vi "_PC_MS_SubVI dataProcess.vi"(7 "Init?(F)":bool, 8 "error in (no error)":errorcluster, 10 "newSigInfo":T1, 11 "Reference":T2) -> (0 "error out":errorcluster, 3 "ydata":sgl[][](array[numeric]))   [LabVIEW 2018]
uses:
  <vilib>/Utility/miscctls.llb/LVPositionTypeDef.ctl
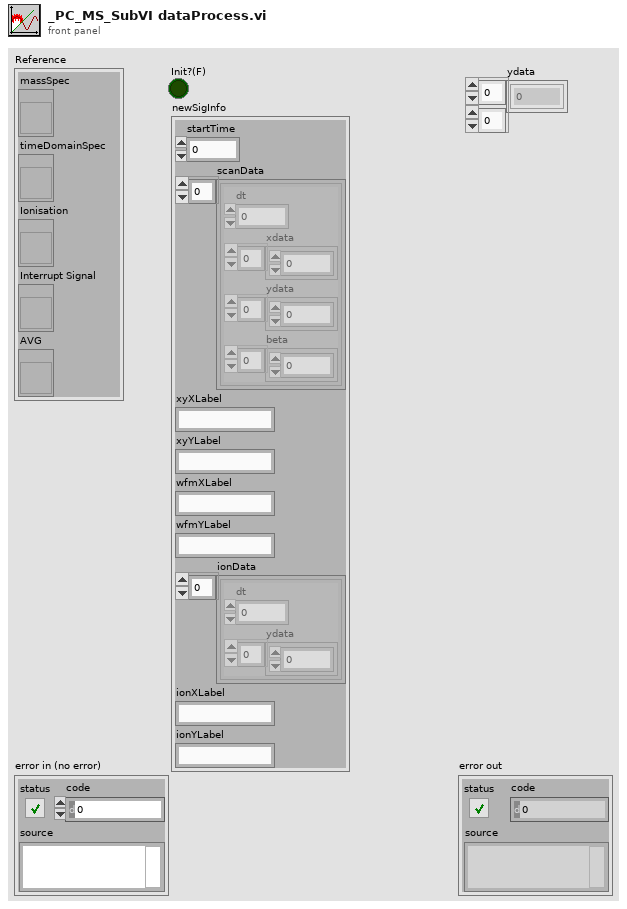
[diagram p1: front panel]
types:
  T1 = cluster{"startTime":dbl, "scanData":cluster{"dt":dbl, "xdata":dbl[], "ydata":sgl[], "beta":dbl[]}[], "xyXLabel":string, "xyYLabel":string, "wfmXLabel":string, "wfmYLabel":string, "ionData":cluster{"dt":dbl, "ydata":sgl[]}[], "ionXLabel":string, "ionYLabel":string}
  T2 = cluster{"massSpec":refnum<vi>, "timeDomainSpec":refnum<vi>, "Ionisation":refnum<vi>, "Interrupt Signal":refnum<vi>, "AVG":refnum<vi>}
  T3 = cluster{"massSpec":refnum<vi>, "timeDomainSpec":refnum<vi>, "Ionisation":refnum<vi>}
  T4 = typedef "LVPositionTypeDef.ctl" = cluster{"Left":i32, "Top":i32}
  T5 = typedef "LVRectTypeDef.ctl" = cluster{"Left":i16, "Top":i16, "Right":i16, "Bottom":i16}
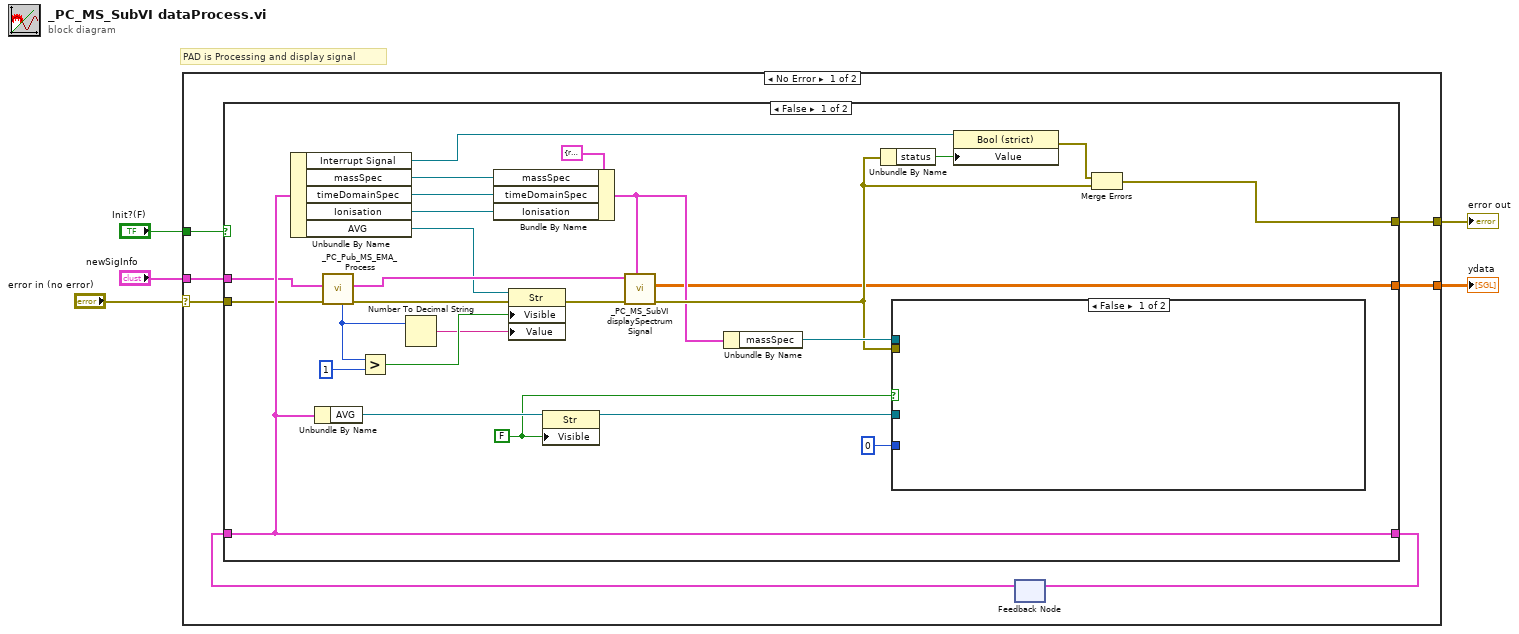
[diagram p0: block diagram]
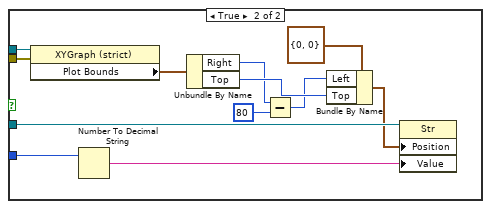
[diagram p2: hidden frame]
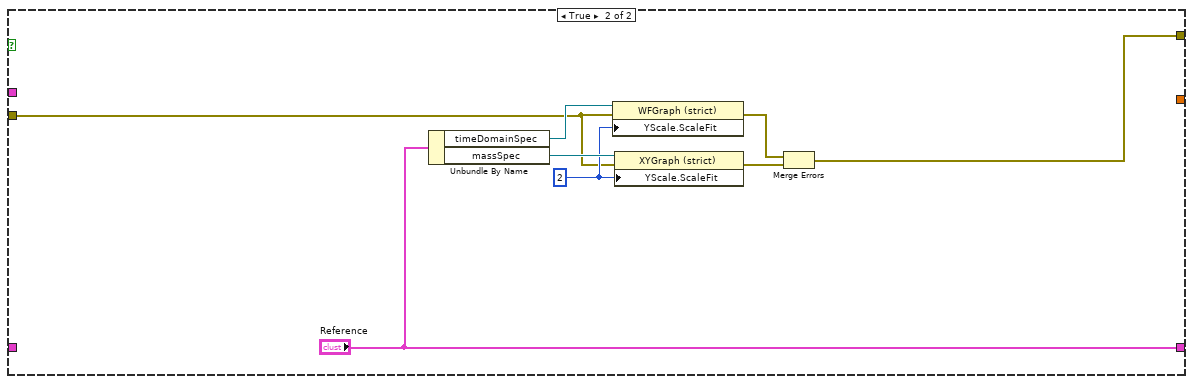
[diagram p3: hidden frame]
diagram:
  # "PAD is Processing and display signal"
  n1 = case shown="No Error" "error in (no error)" {
    selector: "error in (no error)" -> [w6 w60]
    tunnel: "Init?(F)" -> [w12 _]
    tunnel: [w11 w60] -> w4
    tunnel: "newSigInfo" -> [w8 _]
    tunnel: [w7 _] -> w2
    frame No Error {
      n2 = feedback #1() -> (w9:T2)  [unwired: 1 in]
      n3 = case shown="False" w12 {
        tunnel: w9 -> [w34 _]
        tunnel: [w34 "Reference"] -> w10
        tunnel: w8 -> [w22 _]
        tunnel: w6 -> [w20 w53]
        tunnel: [w36 w54] -> w11
        tunnel: [w23 _] -> w7
        frame False {
          w28 = FALSE ("Visible")
          n4 = Unbundle By Name(w34) -> ("Interrupt Signal"=w39:refnum<vi>, "massSpec"=w33:refnum<vi>, "timeDomainSpec"=w30:refnum<vi>, "Ionisation"=w26:refnum<vi>, "AVG"=w18:refnum<vi>)
          n5 = Unbundle By Name(w34) -> ("AVG"=w35:refnum<vi>)
          n6 = call "_PC_Pub_MS_EMA_Process.vi"("error in (no error)"=w20, "SigInfo in"=w22) -> ("error out"=w16:errorcluster, "SigInfo out"=w21:T1, "AVG Items"=w14:u8)  [unwired: 7 in]
          n7 = Greater?(x=w14, y=u8 1) -> (0:w17:bool)
          n8 = Number To Decimal String(number=w14) -> (decimal integer string=w13:string)  [unwired: 1 in]
          n9 = Bundle By Name(cluster=T3 {"massSpec"=refnum, "timeDomainSpec"=refnum, "Ionisation"=refnum}, "massSpec"=w33, "timeDomainSpec"=w30, "Ionisation"=w26) -> (w25:T3)
          n10 = property class="Str"(reference=w18, error in=w16, "Visible"=w17, "Value"=w13) -> (error out=w15:errorcluster)  [unwired: 1 out]
          n11 = property class="Str"(reference=w35, "Visible"=w28) -> (reference out=w37:refnum<vi>)  [unwired: 1 in, 1 out]
          n12 = call "_PC_MS_SubVI displaySpectrumSignal.vi"("graphRefnum in"=w25, "error in (no error)"=w15, "newSigInfo"=w21) -> ("error out"=w29:errorcluster, "ydata"=w23:sgl[][])  [unwired: 7 in]
          n13 = Unbundle By Name(w25) -> ("massSpec"=w32:refnum<vi>)
          n14 = Unbundle By Name(w29) -> ("status"=w38:bool)
          n15 = case shown="False" w28 {
            tunnel: w32 -> [_ w51]
            tunnel: w37 -> [_ w49]
            tunnel: w29 -> [_ w45]
            tunnel: u8 0 ("AVG Items") -> [_ w44]
            frame False {
            }
            frame True {
              n16 = property class="XYGraph (strict)"(reference=w51, error in=w45) -> ("Plot Bounds"=w50:T5)  [unwired: 2 out]
              n17 = Number To Decimal String(number=w44) -> (decimal integer string=w43:string)  [unwired: 1 in]
              n18 = Unbundle By Name(w50) -> ("Right"=w42:i16, "Top"=w47:i16)
              n19 = Subtract(x=w42, y=i16 80) -> (x-y=w40:i16)
              n20 = Bundle By Name(cluster=T4 {"Left"=0, "Top"=0} ("Position"), "Left"=w40, "Top"=w47) -> (w46:T4)
              n21 = property class="Str"(reference=w49, "Position"=w46, "Value"=w43) -> ()  [unwired: 1 in, 2 out]
            }
          }
          n22 = property class="Bool (strict)"(reference=w39, "Value"=w38) -> (error out=w24:errorcluster)  [unwired: 1 in, 1 out]
          n23 = Merge Errors(w24, w29) -> (w36:errorcluster)
        }
        frame True {
          w57 = u8 2 ("Y Scale.Scale Fit")
          n24 = Unbundle By Name("Reference") -> ("timeDomainSpec"=w58:refnum<vi>, "massSpec"=w59:refnum<vi>)
          n25 = property class="WFGraph (strict)"(reference=w58, error in=w53, "YScale.ScaleFit"=w57) -> (error out=w56:errorcluster)  [unwired: 1 out]
          n26 = property class="XYGraph (strict)"(reference=w59, error in=w53, "YScale.ScaleFit"=w57) -> (error out=w55:errorcluster)  [unwired: 1 out]
          n27 = Merge Errors(w56, w55) -> (w54:errorcluster)
        }
      }
      n28 = feedback-in #1(w10) -> ()
    }
    frame Error {
    }
  }
  "error out" <- w4
  "ydata" <- w2
